vi "Py - CsB FL K loop.vi"(6 "Int_array":dbl[](array[numeric]), 7 "python in":refnum<k35>, 8 "error in":errorcluster, 9 "En_array":dbl[](array[numeric]), 10 "Lin":i32, 11 "Z":i32) -> (0 "error out":errorcluster, 2 "Num Iterations":i32, 3 "CsB FL K":dbl, 5 "python out":refnum<k35>)   [LabVIEW 2023]
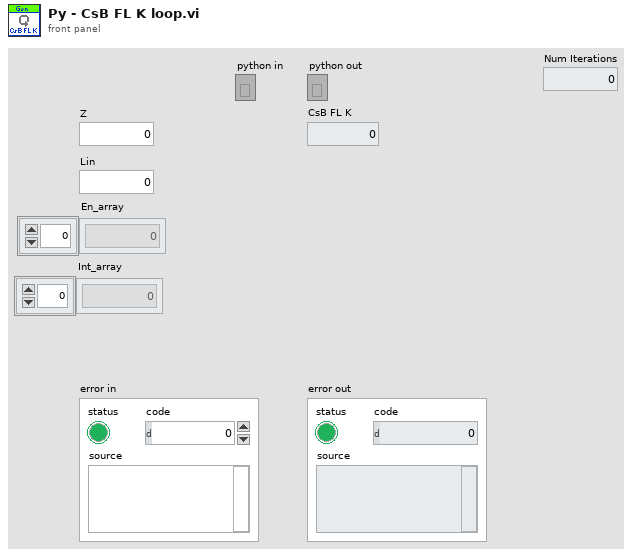
[diagram p1: front panel]
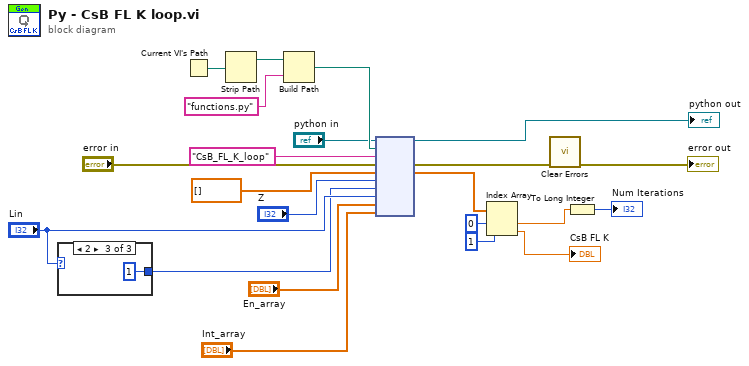
[diagram p0: block diagram]
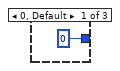
[diagram p2: hidden frame]
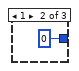
[diagram p3: hidden frame]
diagram:
  n1 = case shown="2" "Lin" {
    tunnel: [0 0 1] -> w1
    frame 0, Default {
    }
    frame 1 {
    }
    frame 2 {
    }
  }
  n2 = Current VI's Path() -> (path=w21:path)
  n3 = Strip Path(path=w21) -> (stripped path=w20:path)  [unwired: 1 out]
  n4 = Build Path(base path=w20, name or relative path="functions.py") -> (appended path=w17:path)
  n5 = node("python in", w17, "CsB_FL_K_loop", "error in", dbl[] [], "Z", w1, "Lin", "En_array", "Int_array") -> (→"python out":refnum<k35>, w8:errorcluster, w14:dbl[])  [unwired: 5 in, 2 out]
  n6 = Index Array(array=w14, index #1=0 ("index"), index #2=1 ("index")) -> (element #1=w10:dbl, element #2=→"CsB FL K":dbl)
  n7 = call <vilib>:"Clear Errors.vi"("error in (no error)"=w8) -> ("error out"=→"error out":errorcluster)  [unwired: 5 in, 1 out]
  n8 = To Long Integer(number=w10) -> (32bit integer=→"Num Iterations":i32)
